vi "MPExxx_conf.vi"(2 "Interlock":bool, 3 "Remote Sense":bool, 4 "error in (no error)":errorcluster, 5 "External Control":bool, 6 "Internal Control":bool=TRUE, 7 "VISA session":refnum<visa-resource-name>) -> (0 "error out":errorcluster, 1 "dup VISA session":refnum<visa-resource-name>)   [LabVIEW 2017]
doc: "This VI form configures the power supply's Remote Sense, Internal Control, External Control and interlock protection. You specify the values for the power supply."
panel:
  # "MAGNA-POWER"
  # "ON"
  # "ON"
  # "ON"
  # "ON"
  # "OFF"
  # "OFF"
  # "OFF"
  # "OFF"
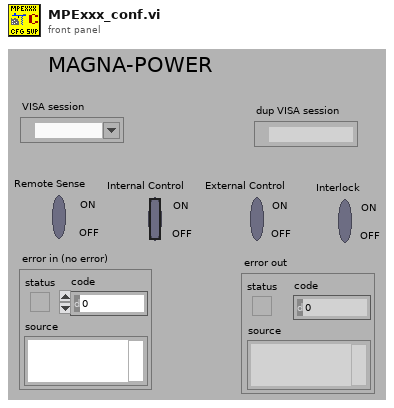
[diagram p1: front panel]
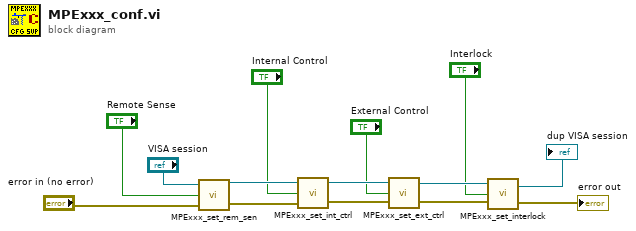
[diagram p0: block diagram]
diagram:
  n1 = call "MPExxx_set_rem_sen.vi"("error in (no error)"="error in (no error)", "Remote Sense"="Remote Sense", "VISA session"="VISA session") -> ("error out"=w14:errorcluster, "dup VISA session"=w9:refnum<visa-resource-name>)
  n2 = call "MPExxx_set_int_ctrl.vi"("error in (no error)"=w14, "Internal Control"="Internal Control", "VISA session"=w9) -> ("error out"=w13:errorcluster, "dup VISA session"=w10:refnum<visa-resource-name>)
  n3 = call "MPExxx_set_ext_ctrl.vi"("error in (no error)"=w13, "External Control"="External Control", "VISA session"=w10) -> ("error out"=w12:errorcluster, "dup VISA session"=w11:refnum<visa-resource-name>)
  n4 = call "MPExxx_set_interlock.vi"("error in (no error)"=w12, "Interlock"="Interlock", "VISA session"=w11) -> ("error out"=→"error out":errorcluster, "dup VISA session"=→"dup VISA session":refnum<visa-resource-name>)
